vi "testSendEvt.vi"(8 "error in (no error)":errorcluster) -> (0 "error out":errorcluster)   [LabVIEW 2018]
doc: "Test the sendEvt.vi."
uses:
  src/TcpServer/TcpServer.lvclass
  <vilib>/addons/_JKI Toolkits/Caraya/classes/Assert/Assert Equal Value_Variant.vi
  <vilib>/addons/_JKI Toolkits/Caraya/classes/Test/Test.lvclass
  <vilib>/addons/_JKI Toolkits/Caraya/classes/Assert/Assert.lvclass
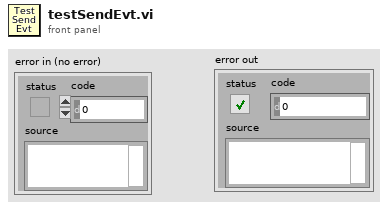
[diagram p1: front panel]
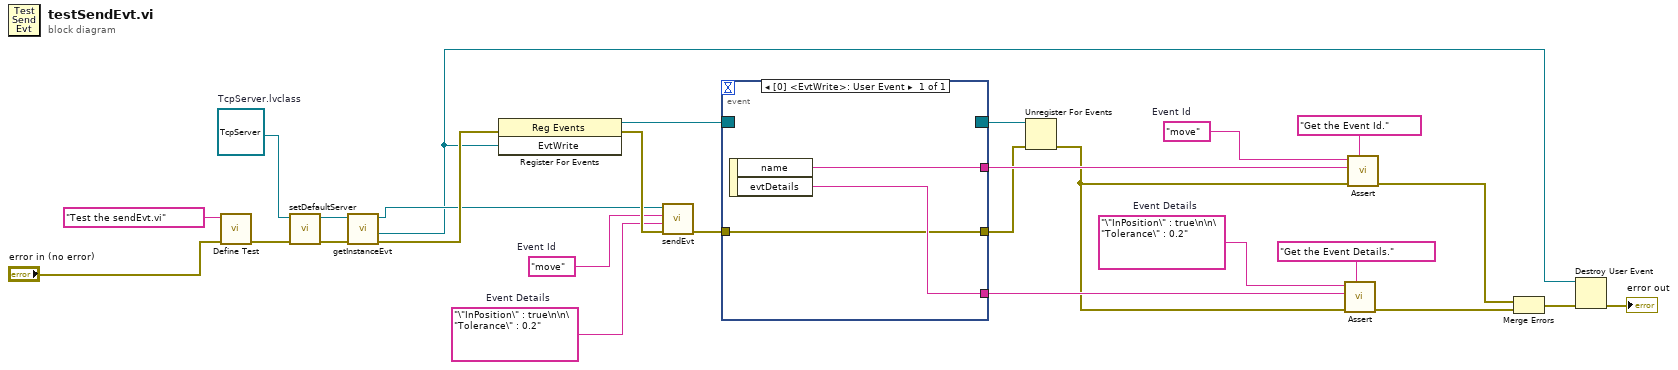
[diagram p0: block diagram]
diagram:
  w1 = "\"InPosition\" : true\n\n\"Tolerance\" : 0.2"  # Event Details
  w2 = "move"  # Event Id
  w3 = "\"InPosition\" : true\n\n\"Tolerance\" : 0.2"  # Event Details
  w4 = "move"  # Event Id
  w24 = refnum<class "TcpServer.lvclass"> refnum  # TcpServer.lvclass
  n1 = call <vilib>:"Define Test.vi"("error in (no error)"="error in (no error)", "Label (VI Title)"="Test the sendEvt.vi") -> ("error out"=w26:errorcluster)  [unwired: 9 in]
  n2 = call "setDefaultServer.vi"("error in (no error)"=w26, "TcpServer.lvclass"=w24) -> ("error out"=w7:errorcluster, "tcpServer out"=w8:refnum<class "TcpServer.lvclass">)  [unwired: 8 in]
  n3 = call "getInstanceEvt.vi"("error in (no error)"=w7, "tcpServer in"=w8) -> ("error out"=w9:errorcluster, "EvtWrite"=w5:refnum<user-event>, "tcpServer out"=w6:refnum<class "TcpServer.lvclass">)  [unwired: 6 in, 1 out]
  n4 = register-events(error in=w9, w5) -> (reference out=w23:refnum<event-registration>, error out=w22:errorcluster)  [unwired: 1 in]
  n5 = call "sendEvt.vi"("error in (no error)"=w22, "Event Details"=w3, "Event Id"=w4, "tcpServer out"=w6) -> ("error out"=w14:errorcluster)  [unwired: 7 in]
  n6 = event shown="[0] <EvtWrite>: User Event" {
    selector: w23 -> [_]
    dyn-events: [_] -> w13
    timeout: _ -> [_]
    tunnel: [w30] -> w19
    tunnel: [w29] -> w17
    tunnel: w14 -> [w28]
    tunnel: [w28] -> w12
    event User Event {
      n7 = event-data() -> ("name"=w29:string, "evtDetails"=w30:string)  [unwired: 1 in]
    }
  }
  n8 = Unregister For Events(event registration refnum=w13, error in=w12) -> (error out=w11:errorcluster)
  n9 = call-poly <vilib>:"Assert.vi"("Label"="Get the Event Details.", "error in (no error)"=w11, "Y"=w19, "X"=w1) -> ("error out"=w16:errorcluster)  [unwired: 7 in]
  n10 = call-poly <vilib>:"Assert.vi"("Label"="Get the Event Id.", "error in (no error)"=w11, "Y"=w17, "X"=w2) -> ("error out"=w15:errorcluster)  [unwired: 7 in]
  n11 = Merge Errors(w15, w16) -> (w21:errorcluster)
  n12 = Destroy User Event(user event=w5, error in=w21) -> (error out=→"error out":errorcluster)
